vi "qSEP_Hex.vi"(0 "System no.":i32=1 min=1 max=4 step=1, 2 "Axes to query":string[](array[string]), 3 "Without axes?":bool, 5 "error in":errorcluster, 6 "Parameter no. (hex)":u32[](array[numeric]) format="%.0x") -> (14 "Parameter string":string[](array[string]), 19 "error out":errorcluster)   [LabVIEW 2026]
doc: "Returns parameter string from non-volatile memory for queried axis and hex. parameter number. Old VI - please use SEP?.vi instead.\n\nE-710: See E-710 GCS DLL manual for a detailed list of available parameter numbers. Without axes? can be TRUE and will return all available parameter for all axes.\nE-761: See E-761 GCS DLL manual for a detailed list of available parameter numbers. Without axes? can be TRUE and will return all available parameter for all axes."
uses:
  Communication/Global1.vi
panel:
  # "Returns Eprom parameter string for queried axis and hex. parameter number. Old VI - please use \nSEP?.vi instead."
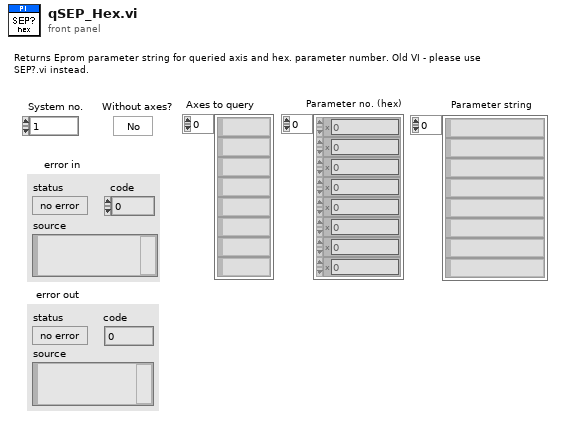
[diagram p1: front panel]
types:
  T1 = typedef "Syntax.ctl" = enum16{"GCS 1.0", "GCS 2.0", "GCS 3.0"}
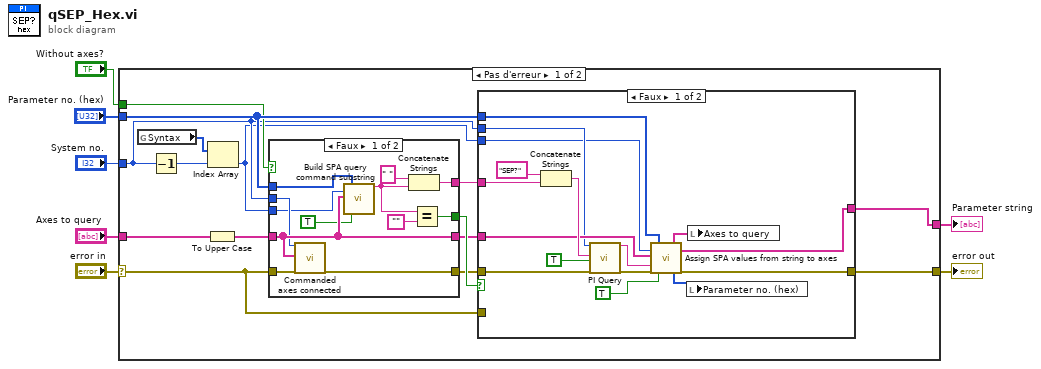
[diagram p0: block diagram]
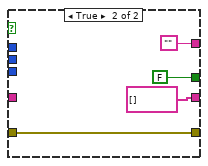
[diagram p2: hidden frame]
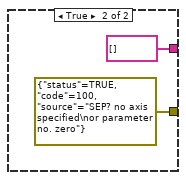
[diagram p3: hidden frame]
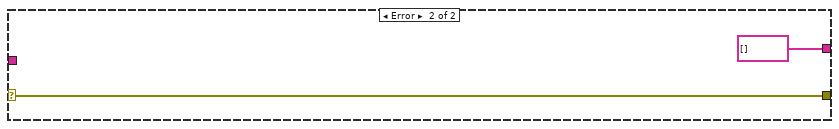
[diagram p4: hidden frame]
diagram:
  n1 = case shown="Pas d'erreur" "error in" {
    selector: "error in" -> [w8 w57]
    tunnel: "Axes to query" -> [w22 _]
    tunnel: "System no." -> [w10 _]
    tunnel: "Parameter no. (hex)" -> [w16 _]
    tunnel: [w19 w57] -> w4
    tunnel: [w17 string[] [] ("Parameter strings")] -> w3
    tunnel: "Without axes?" -> [w14 _]
    frame No Error {
      n2 = global read "Global1.vi" "Syntax"() -> (w11:T1[])
      n3 = Decrement(x=w10) -> (x-1=w12:i32)
      n4 = To Upper Case(1:w22) -> (0:w20:string[])
      n5 = Index Array(array=w11, index=w12) -> (element=w9:T1)
      n6 = case shown="Faux" w14 {
        tunnel: [w27 "" ("Command substring")] -> w21
        tunnel: w20 -> [w29 _]
        tunnel: [w33 FALSE] -> w18
        tunnel: w16 -> [w32 _]
        tunnel: [w29 string[] []] -> w15
        tunnel: w8 -> [w31 w36]
        tunnel: [w30 w36] -> w13
        tunnel: w10 -> [w28 _]
        tunnel: w9 -> [w24 _]
        frame False {
          n7 = call "Commanded axes connected.vi"("System no."=w28, "Commanded axes"=w29, "error in"=w31) -> ("error out"=w30:errorcluster)  [unwired: 1 in, 15 out]
          n8 = call "Build SPA query command substring.vi"("Syntax"=w24, "Axes to query"=w29, "Parameter number (hex)"=w32, "Parameter no. format \n(Decimal: FALSE)"=TRUE ("Parameter no. format \n(Decimal: FALSE)")) -> ("Command substring"=w26:string)  [unwired: 1 in, 14 out]
          n9 = Concatenate Strings(" " ("Substring"), w26) -> (w27:string)
          n10 = Equal?(x=w26, y="" ("x")) -> (x = y?=w33:bool)
        }
        frame True {
        }
      }
      n11 = case shown="Faux" w18 {
        tunnel: w8 -> [_ _]
        tunnel: w21 -> [w51 _]
        tunnel: w15 -> [w50 _]
        tunnel: w10 -> [w42 _]
        tunnel: w16 -> [w43 _]
        tunnel: [w49 errorcluster {"status"=TRUE, "code"=100, "source"="SEP? no axis specified\nor parameter no. zero"} ("error out")] -> w19
        tunnel: [w48 string[] [] ("Parameter strings")] -> w17
        tunnel: w13 -> [w47 _]
        tunnel: w9 -> [w41 _]
        frame False {
          n12 = Concatenate Strings("SEP?", w51) -> (w52:string)
          n13 = call "PI Query.vi"("System no."=w42, "String to send"=w52, "Attach termination char.?"=TRUE ("Attach Linefeed?"), "error in"=w47) -> ("String read"=w39:string, "error out"=w40:errorcluster)  [unwired: 3 in, 11 out]
          n14 = call "Assign SPA values from string to axes.vi"("Syntax"=w41, "Queried axes"=w50, "Input string"=w39, "error in"=w40, "Parameter no. (hex)"=w43, "Parameter no. format \n(Decimal: FALSE)"=TRUE ("Parameter no. format \n(Decimal: FALSE)")) -> ("Queried axes out"=w46:string[], "Parameter no. (hex) out"=w45:u32[], "Parameter strings"=w48:string[], "error out"=w49:errorcluster)  [unwired: 1 in, 9 out]
          n15 = local write "Parameter no. (hex)"(w45) -> ()
          n16 = local write "Axes to query"(w46) -> ()
        }
        frame True {
        }
      }
    }
    frame Error {
    }
  }
  "error out" <- w4
  "Parameter string" <- w3
